vi "动子12侧CT内容.vi"() -> (0 "Frist ColData":string, 1 "UpDateData":string[](array[string]), 2 "tablename":string, 3 "UpDateCol":string[](array[string]))   [LabVIEW 2017]
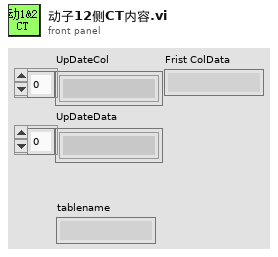
[diagram p1: front panel]
types:
  T1 = typedef "动子1&2CT操作选项.ctl" = enum16{"初始化", "出料轴接料", "投掷出料区", "获取寄存器", "更新等待CT"}
  T2 = typedef "data格式选项.ctl" = enum16{"生成格式", "加载格式"}
  T3 = typedef "缓存操作选项.ctl" = enum16{"初始化", "量测缓存写入", "前侧获取索引", "后侧获取索引", "前侧更新索引", "后侧更新索引", "获取寄存器"}
  T4 = typedef "Data_CT索引操作缓存.ctl" = cluster{"当前data行索引":i32[], "data更新获取索引":T5, "前排提取行号":string, "后排提取行号":string, "当前量测站行号":string, "当前_datetime":string, "量测站操作table缓存":string[], "前排提取_datetime":string, "后排提取_datetime":string}
  T5 = typedef "data更新获取索引.ctl" = cluster{"data更新索引":i32, "前侧获取索引":i32, "后侧获取索引":i32}
  T6 = typedef "表头集合.ctl" = cluster{"product信息":T7, "CT信息":T8, "ER信息":T9, "IOT信息":T10}
  T7 = typedef "product信息.ctl" = cluster{"product表头整合":string[], "量测部分表头":string[], "前侧贴合表头":string[], "后侧贴合表头":string[]}
  T8 = typedef "CT信息.ctl" = cluster{"CT表头整合":string[], "量测CT":string[], "动子1_2CT":string[], "动子3_4CT":string[]}
  T9 = typedef "ER信息.ctl" = cluster{"ER表头整合":string[]}
  T10 = typedef "IOT信息.ctl" = cluster{"IOT表头整合":string[]}
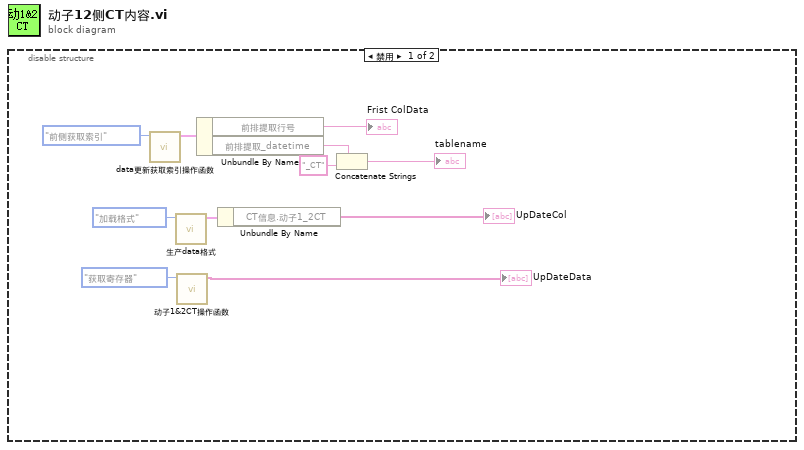
[diagram p0: block diagram]
diagram:
  n1 = disable-structure shown="禁用" {
    frame Disabled {
      n2 = call "data更新获取索引操作函数.vi"("缓存操作选项"=缓存操作选项."前侧获取索引") -> ("Data_CT索引操作缓存"=w10:T4)  [unwired: 9 in, 1 out]
      n3 = call "生产data格式.vi"("data格式选项"=data格式选项."加载格式") -> ("表头格式"=w8:T6)  [unwired: 10 in]
      n4 = call "动子1&2CT操作函数.vi"("CT操作选项"=动子1&2CT操作选项."获取寄存器") -> ("CT集合"=→"UpDateData":string[])  [unwired: 9 in, 1 out]
      n5 = Unbundle By Name(w10) -> ("前排提取行号"=→"Frist ColData":string, "前排提取_datetime"=w3:string)
      n6 = Unbundle By Name(w8) -> ("CT信息.动子1_2CT"=→"UpDateCol":string[])
      n7 = Concatenate Strings(w3, "_CT" ("字符串")) -> (→"tablename":string)
    }
    frame Enabled {
    }
  }
